vi "Msg.vi"(7 "Actor in":refnum<class "Actor.lvclass">, 11 "Has Destroyed Msg in":refnum<class "Has Destroyed Msg.lvclass">) -> (0 "Error out":errorcluster, 5 "Actor out":refnum<class "Actor.lvclass">)   [LabVIEW 2020, in "jettl.lvlib" / "Has Destroyed Msg.lvlib" / "Has Destroyed Msg.lvclass"]
uses:
  Has Destroyed Msg.lvclass
  Actor/Actor/Actor.lvclass
  Has Destroyed/Has Destroyed.lvclass
  Has Destroyed Msg.lvclass/Has Destroyed Msg.ctl
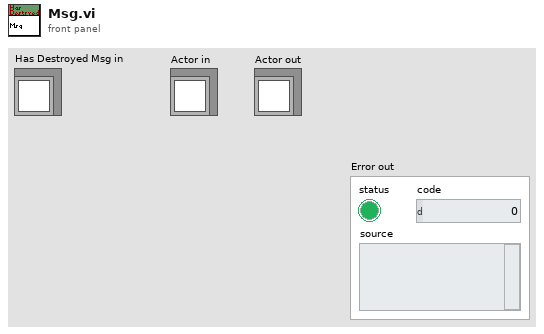
[diagram p1: front panel]
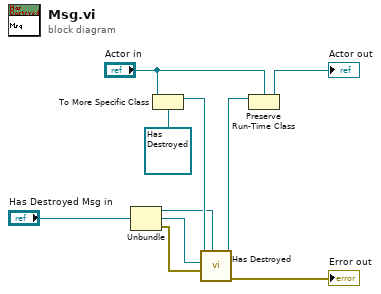
[diagram p0: block diagram]
diagram:
  n1 = Unbundle "Unbundle"("Has Destroyed Msg in") -> (w3:refnum<class "Sender.lvclass">, w4:refnum<class "Actor.lvclass">, w2:errorcluster)
  n2 = To More Specific Class(target class=refnum<class "Has Destroyed.lvclass"> refnum ("jettl.lvlib:jettl Msg Last Ack Creator Queue.lvlib:jettl Msg Last Ack Creator Queue.lvclass"), reference="Actor in") -> (specific class reference=w6:refnum<class "Has Destroyed.lvclass">)  [unwired: 1 in, 1 out]
  n3 = call-dynamic "Has Destroyed.vi"("Sender"=w3, "Error"=w2, "Actor"=w4, "Has Destroyed in"=w6) -> ("Error out"=→"Error out":errorcluster, "Has Destroyed out"=w5:refnum<class "Has Destroyed.lvclass">)  [unwired: 6 in]
  n4 = Preserve Run-Time Class(object in=w5, 2:"Actor in") -> (object out=→"Actor out":refnum<class "Actor.lvclass">)  [unwired: 1 in, 1 out]
